vi "Log Status Update.vi"(8 "error in (no error)":errorcluster, 10 "Status":string, 11 "Mag Lab Measure Interface in":refnum<class "Mag Lab Measure UI.lvclass">) -> (0 "error out":errorcluster, 3 "Mag Lab Measure Interface out":refnum<class "Mag Lab Measure UI.lvclass">)   [LabVIEW 2015, in "Mag Lab Measure UI.lvclass"]
uses:
  Mag Lab Measure UI.lvclass
  Mag Lab Measure UI.lvclass/Mag Lab Measure UI.ctl
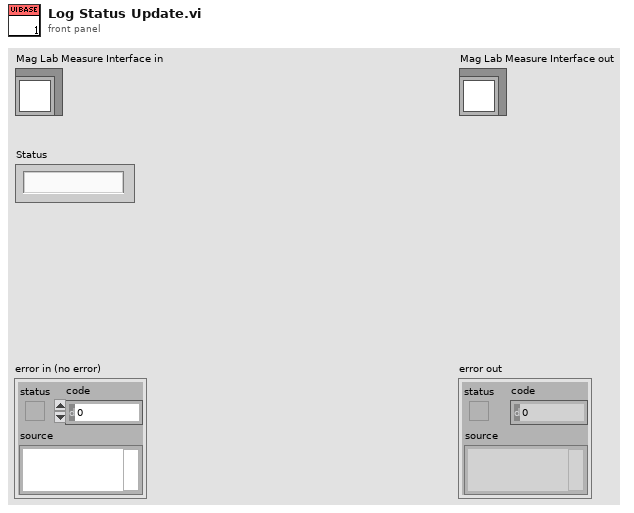
[diagram p1: front panel]
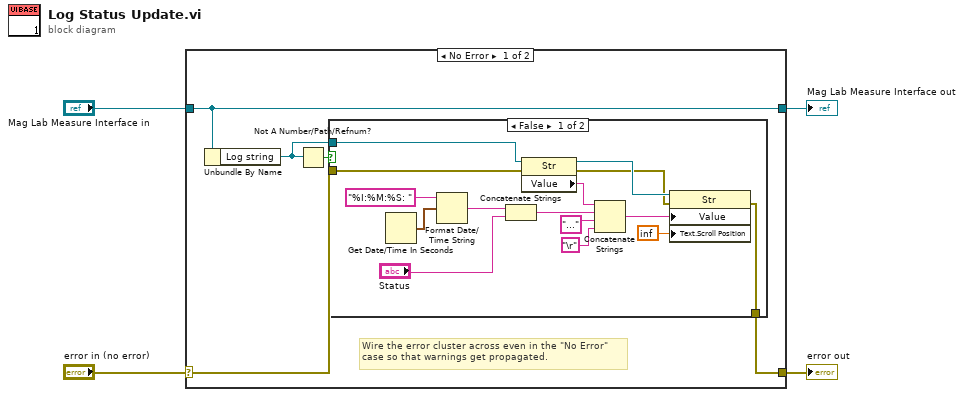
[diagram p0: block diagram]
diagram:
  n1 = case shown="No Error" "error in (no error)" {
    selector: "error in (no error)" -> [w6 w27]
    tunnel: [w5 w27] -> w3
    tunnel: [w9 w26] -> w1
    tunnel: "Mag Lab Measure Interface in" -> [w9 w26]
    frame No Error {
      # "Wire the error cluster across even in the \"No Error\"\ncase so that warnings get propagated."
      n2 = Unbundle By Name(w9) -> ("Log string"=w7:refnum<vi>)
      n3 = Not A Number/Path/Refnum?(number/path/refnum=w7) -> (NaN/Path/Refnum?=w8:bool)
      n4 = case shown="False" w8 {
        tunnel: w7 -> [w13 _]
        tunnel: w6 -> [w12 w25]
        tunnel: [w10 w25] -> w5
        frame False {
          n5 = Get Date/Time In Seconds() -> (seconds since 1Jan1904=w22:timestamp)
          n6 = Format Date/Time String(time format string (%c)="%I:%M:%S: ", seconds (now)=w22) -> (date/time string=w24:string)  [unwired: 1 in]
          n7 = Concatenate Strings(w24, "Status") -> (w15:string)
          n8 = property class="Str"(reference=w13, error in=w12) -> (reference out=w17:refnum<vi>, error out=w11:errorcluster, "Value"=w18:string)
          n9 = Concatenate Strings(w18, w15, "..." ("string"), "\r") -> (w16:string)
          n10 = property class="Str"(reference=w17, error in=w11, "Value"=w16, "Text.Scroll Position"=inf) -> (error out=w10:errorcluster)  [unwired: 1 out]
        }
        frame True {
        }
      }
    }
    frame Error {
    }
  }
  "error out" <- w3
  "Mag Lab Measure Interface out" <- w1
